vi "Get Transfer Type.vi"(8 "error in":errorcluster, 11 "label ref in":T2 format="%.0x") -> (0 "error out":errorcluster, 2 "transfer type":T1, 3 "label ref out":T2 format="%.0x")   [LabVIEW 2020, in "ARINC 429 Scripting.lvlib"]
uses:
  ARINC 429 Scripting.lvlib
  <vilib>/NI VeriStand/Custom Device API/Custom Device Item Ref.ctl
  Shared/Transfer Type.ctl
  Constants.vi
  <vilib>/NI VeriStand/Custom Device API/Get Item Property (U16).vi
  <vilib>/NI VeriStand/Custom Device API/Custom Device API.lvlib
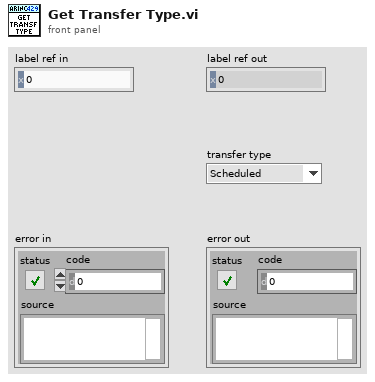
[diagram p1: front panel]
types:
  T1 = typedef "Transfer Type.ctl" = enum16{"Scheduled", "Acyclic", "Block", "Strobe"}
  T2 = typedef "Custom Device API.lvlib/Custom Device Item Ref.ctl" = u64
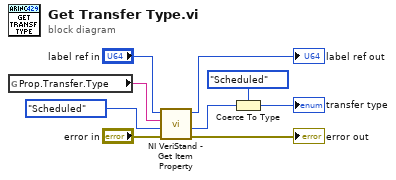
[diagram p0: block diagram]
diagram:
  n1 = global read "Constants.vi" "Prop.Transfer.Type"() -> (w7:string)
  n2 = call-poly <vilib>:"NI VeriStand - Get Item Property.vi"("error in (no error)"="error in", "Default Value"=Transfer_Type."Scheduled" ("transfer type"), "Property Name"=w7, "Item Ref in"="label ref in") -> ("error out"=→"error out":errorcluster, "Value"=w2:u16, "Item Ref out"=→"label ref out":T2)  [unwired: 4 in, 1 out]
  n3 = Coerce To Type(0:w2, 1:Transfer_Type."Scheduled" ("transfer type")) -> (2:→"transfer type":T1)
